vi "SIMPLE 2D Sweep -MAIN.vi"() -> ()   [LabVIEW 2025]
doc: "This is a program providing a single inclusive measurement platform in LabVIEW for every 2D sweep created by Pratap Chandra Adak."
uses:
  TYPE DEFS/S2DS_Instrument Info.ctl
  TYPE DEFS/S2DS_Instrument parameters.ctl
  TYPE DEFS/S2DS_All Channel Parameters.ctl
  TYPE DEFS/S2DS_WC info.ctl
  TYPE DEFS/S2DS_Single WC info.ctl
  TYPE DEFS/S2DS_RC info.ctl
  TYPE DEFS/S2DS_Single RC info.ctl
  TYPE DEFS/S2DS_DAC info new.ctl
  TYPE DEFS/S2DS_Single DC info.ctl
  TYPE DEFS/S2DS_Array Inst Info.ctl
  TYPE DEFS/S2DS_Sweep Info.ctl
  TYPE DEFS/S2DS_Display info.ctl
  TYPE DEFS/S2DS_Data saving info.ctl
  TYPE DEFS/S2DS_Port lists.ctl
  TYPE DEFS/S2DS_Timer.ctl
  TYPE DEFS/S2DS_WCFromFileInfo.ctl
  TYPE DEFS/S2DS_PlotInfo.ctl
  TYPE DEFS/S2DS_PlotCluster.ctl
  <vilib>/Utility/error.llb/Three Button Dialog.vi
panel:
  in  "Pause":bool
  in  "Edit Instrument?":bool
  in  "Quit sweep":bool
  out "?":string=" ( : )"
  in  "Set initial settings":bool
  out "Save location:":path
  out "Prameter error":string
  in  "Tab Control Y":enum32{"Parameters", "Additional"}(tab) caption="B(kUnit)"
  in  "Y Min":dbl caption="Min end"
  in  "Y Max":dbl=1.0 caption="Max end"
  in  "Y Bin size":dbl=0.001 caption="Data bin  size"
  in  "Y Step":dbl=0.001 caption="Ramp step size"
  in  "Y Rate up":dbl=0.1 caption="Rate up/min"
  in  "Y Rate down":dbl=0.1 caption="Rate down/min"
  in  "Y Stop at":u16(ring)=1 items=["Continue", "Stop at end", "Stop at stoppage"]
  in  "Y Skipping":u64 caption="skipping"
  in  "Y Stoppage":dbl caption="Stoppage"
  in  "Ramp Y":bool
  in  "Take data 2":u16(ring) caption="Take data" items=["in both direction", "in up direction only", "in down direction only"]
  in  "Reset skipped Y":bool
  out "Y reached":i32 caption="Reached"
  in  "Tab Control X":enum32{"Parameters", "Additional"}(tab) caption="A(TUnit)"
  in  "X Step":dbl=0.001 caption="Ramp step size"
  in  "X Rate up":dbl=0.1 caption="Rate up/min"
  in  "X Rate down":dbl=0.1 caption="Rate down/min"
  in  "X Bin size":dbl=0.001 caption="Data bin  size"
  in  "X Max":dbl=1.0 caption="Max end"
  in  "X Min":dbl caption="Min end"
  in  "Reset skipped X":bool
  in  "X Stop at":u64(ring) items=["Continue", "Stop at end", "Stop at stoppage"]
  in  "X Skipping":u64 caption="skipping"
  in  "X Stoppage":dbl caption="Stoppage"
  in  "Ramp X":bool
  in  "Take data":u16(ring) items=["in both direction", "in up direction only", "in down direction only"]
  out "X reached":i32 caption="Reached"
  in  "Hide control panel":bool
  in  "Read array instruments":bool
  in  "WC calculation":bool
  in  "Time save?":bool
  in  "Script On?":bool
  in  "Sweep":bool
  in  "Ramping":bool
  in  "Y sweep direction":bool=TRUE caption="B"
  in  "X sweep direction":bool=TRUE caption="A"
  in  "Scan type":u16(ring) items=["WC values from file", "1D Sweep in A(TUnit)", "1D Sweep in B(kUnit)", "2D Sweep in A(TUnit) within B(kUnit)", "2D Sweep in B(kUnit) within A(TUnit)"]
  out "R12":dbl caption="R9( Unit)"
  out "R13":dbl caption="R10( Unit)"
  out "X :":dbl caption="Index"
  out "Y :":dbl caption="A(TUnit)"
  out "R0":dbl caption="B(kUnit)"
  out "R1":dbl caption="R(Unit)"
  out "R2":dbl caption="Freq(Hz)"
  out "R3":dbl caption="V(V)"
  out "R4":dbl caption="R1(ohmm)"
  out "R5":dbl caption="A( Unit)"
  out "R6":dbl caption="A( Unit)"
  out "R7":dbl caption="A( Unit)"
  out "R8":dbl caption="R7( Unit)"
  out "R9":dbl caption="R8( Unit)"
  out "R10":dbl caption="R9( Unit)"
  out "R11":dbl caption="R10( Unit)"
  in  "Refresh inst info":bool
  out "Buffer length:":i32
  in  "Save now to file?":bool
  in  "Clear Buffer?":bool
  in  "Auto color":bool=TRUE
  in  "Change color?":bool
  in  "Clear plot?":bool
  in  "View Plot?":bool=TRUE
  in  "Update plot":bool=TRUE
  in  "Send email":bool
  in  "Timeout":u16=60 min=1 step=1
  in  "Export Data":bool
  in  "External control":bool
  in  "Y axis":u16(ring) items=["Index", "A(TUnit)", "B(kUnit)", "R(Unit)"]
  in  "X axis":u16(ring) items=["Index", "A(TUnit)", "B(kUnit)", "R(Unit)"]
  out "XY Graph":T1(graph) caption="Pratap"
  in  "Timer reset?":bool
  in  "Clear error?":bool
  out "Progress":i32(slide) scale=0.0..100.0
  out "Remaining time: :":string
  out "Elapsed time:":string
  out "Status":string="Back panel not set"
  # "SIMPLE 2D SWEEP (v10.3.10) ..."
  # "S"
  # "VS"
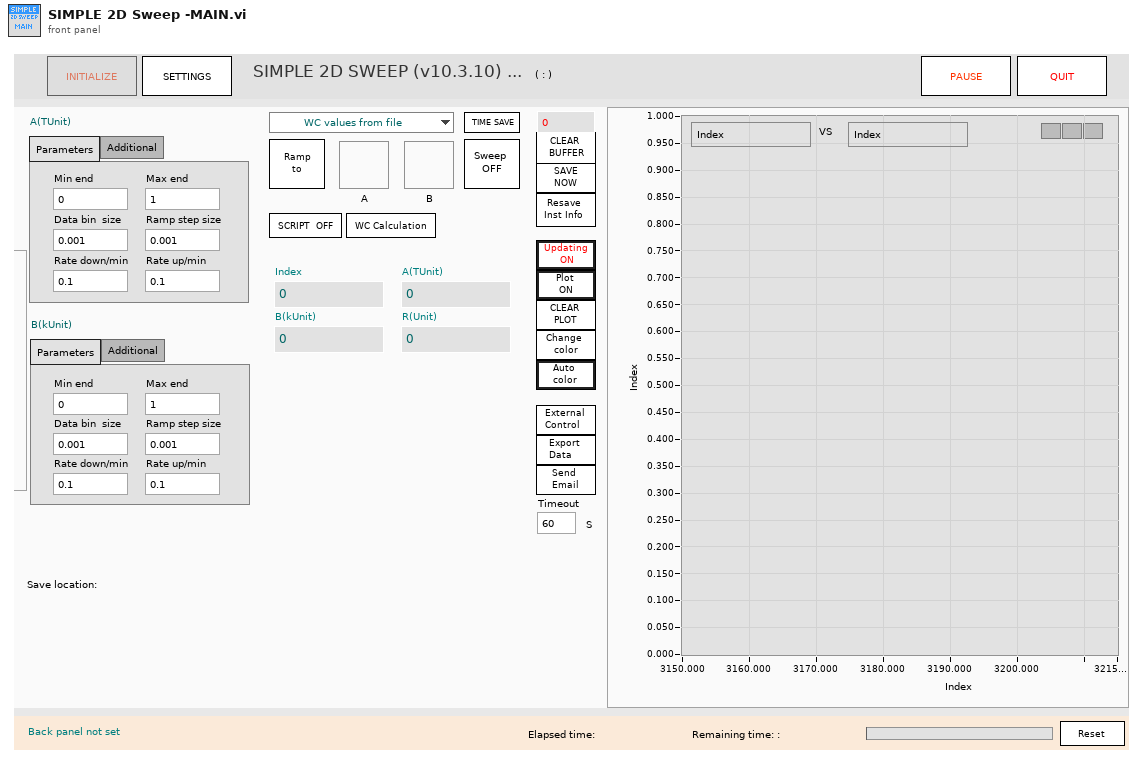
[diagram p1: front panel]
types:
  T1 = cluster{"Plot X array":dbl[], "Plot Z array":dbl[]}[]
  T2 = enum8{"Enabled", "Disabled", "Disabled and Grayed Out"}
  T3 = typedef "S2DS_Data saving info.ctl" = cluster{"File path":path, "Header":string, "File name":string, "False channel":string[][], "Channel names":string[], "Buffer size":i32, "Format":string}
  T4 = typedef "S2DS_Display info.ctl" = cluster{"WCl names with units":string[], "RC  names with units":string[], "DC  names with units":string[], "AC names with units":string[], "Indicator captions":string[], "Graph channels":string[], "Channel numbers":i32[], "User info":string}
  T5 = typedef "S2DS_All Channel Parameters.ctl" = cluster{"WC info list":T6, "RC info list":T8, "DC Info list":T10, "Array instrument info":T12, "Scan parameters":T13, "Parsed Formula Node":cluster{"Y Values":dbl[][], "Tables":i32[][][], "Variables input decode":i32[], "Variables output decode":i32[]}, "formula (in)":string}
  T6 = typedef "S2DS_WC info.ctl" = T7[]
  T7 = typedef "S2DS_Single WC info.ctl" = cluster{"Instrument identifier":string, "Write channel parameters":dbl[], "Name":string, "Unit":string}
  T8 = typedef "S2DS_RC info.ctl" = T9[]
  T9 = typedef "S2DS_Single RC info.ctl" = cluster{"Instrument identifier":string, "Factor":dbl, "Averaging":i32, "Wait (ms)":i32, "Unit":string, "Name":string}
  T10 = typedef "S2DS_DAC info new.ctl" = T11[]
  T11 = typedef "S2DS_Single DC info.ctl" = cluster{"Operation identifier":string, "DC parameters":dbl[], "U":i32, "V":i32, "Name":string, "Unit":string}
  T12 = typedef "S2DS_Array Inst Info.ctl" = cluster{"Instrument identifier":string, "Ports and units":string[][], "Factors":dbl[]}
  T13 = typedef "S2DS_Sweep Info.ctl" = cluster{"X min":ext, "X max":dbl, "Y min":dbl, "Y max":dbl, "X bin size":dbl, "Y bin size":dbl, "X stop at":dbl, "Y stop at":dbl, "X skip":u64, "Y skip":u64, "Current X":dbl, "Current Y":dbl, "X reached":i32, "Y reached":i32, "X target":dbl, "Y target":dbl, "Sweep ON?":bool, "X sweep direction":bool, "Y sweep direction":bool, "Determine X?":bool, "Determine Y?":bool, "X sweep over?":bool, "Y sweep over?":bool, "Scan type":i32, "X stopping":i32, "Y stopping":i32, "X Y Channel":u16[], "X data taking":u16, "Y data taking":u16}
  T14 = typedef "S2DS_Instrument Info.ctl" = cluster{"Instrument parameters":T15[], "DAQ Tasks":refnum<k21>[], "Total Instrument List":string[], "read inst \nVI Refnum":refnum<vi>, "type specifier Edit instruments VI Refnum":refnum<vi>, "type specifier write instrument VI Refnum (for type only)":refnum<vi>, "User instrument list":string[]}
  T15 = typedef "S2DS_Instrument parameters.ctl" = cluster{"VISA Address":refnum<visa-resource-name>, "GPIB/TCP Address":string, "String 1":string, "String 2":string, "Boolean 1":bool, "Boolean 2":bool, "Int 1":i32, "Int 2":i32, "Double 1":dbl, "Double 2":dbl}
  T16 = typedef "S2DS_Port lists.ctl" = cluster{"Write ports":string[], "Read ports":string[], "FC channels":string[][]}
  T17 = typedef "S2DS_PlotInfo.ctl" = cluster{"Plot data array":T18, "Number of curve":i32, "Present curve number XZ":i32}
  T18 = typedef "S2DS_PlotCluster.ctl" = cluster{"Plot i array":dbl[][]}[]
  T19 = typedef "S2DS_WCFromFileInfo.ctl" = cluster{"Next line to read":i32, "Next point in array":i32, "File path":path, "Data to write":dbl[][], "Read offset":i32, "Total line":i32}
  T20 = typedef "S2DS_Timer.ctl" = cluster{"Initial time ":i32, "Total step":i32, "Step completed":i32}
  T21 = cluster{"Y Values":dbl[][], "Tables":i32[][][], "Variables input decode":i32[], "Variables output decode":i32[]}
  T22 = cluster{"Plot X array":dbl[], "Plot Z1 array":dbl[]}[]
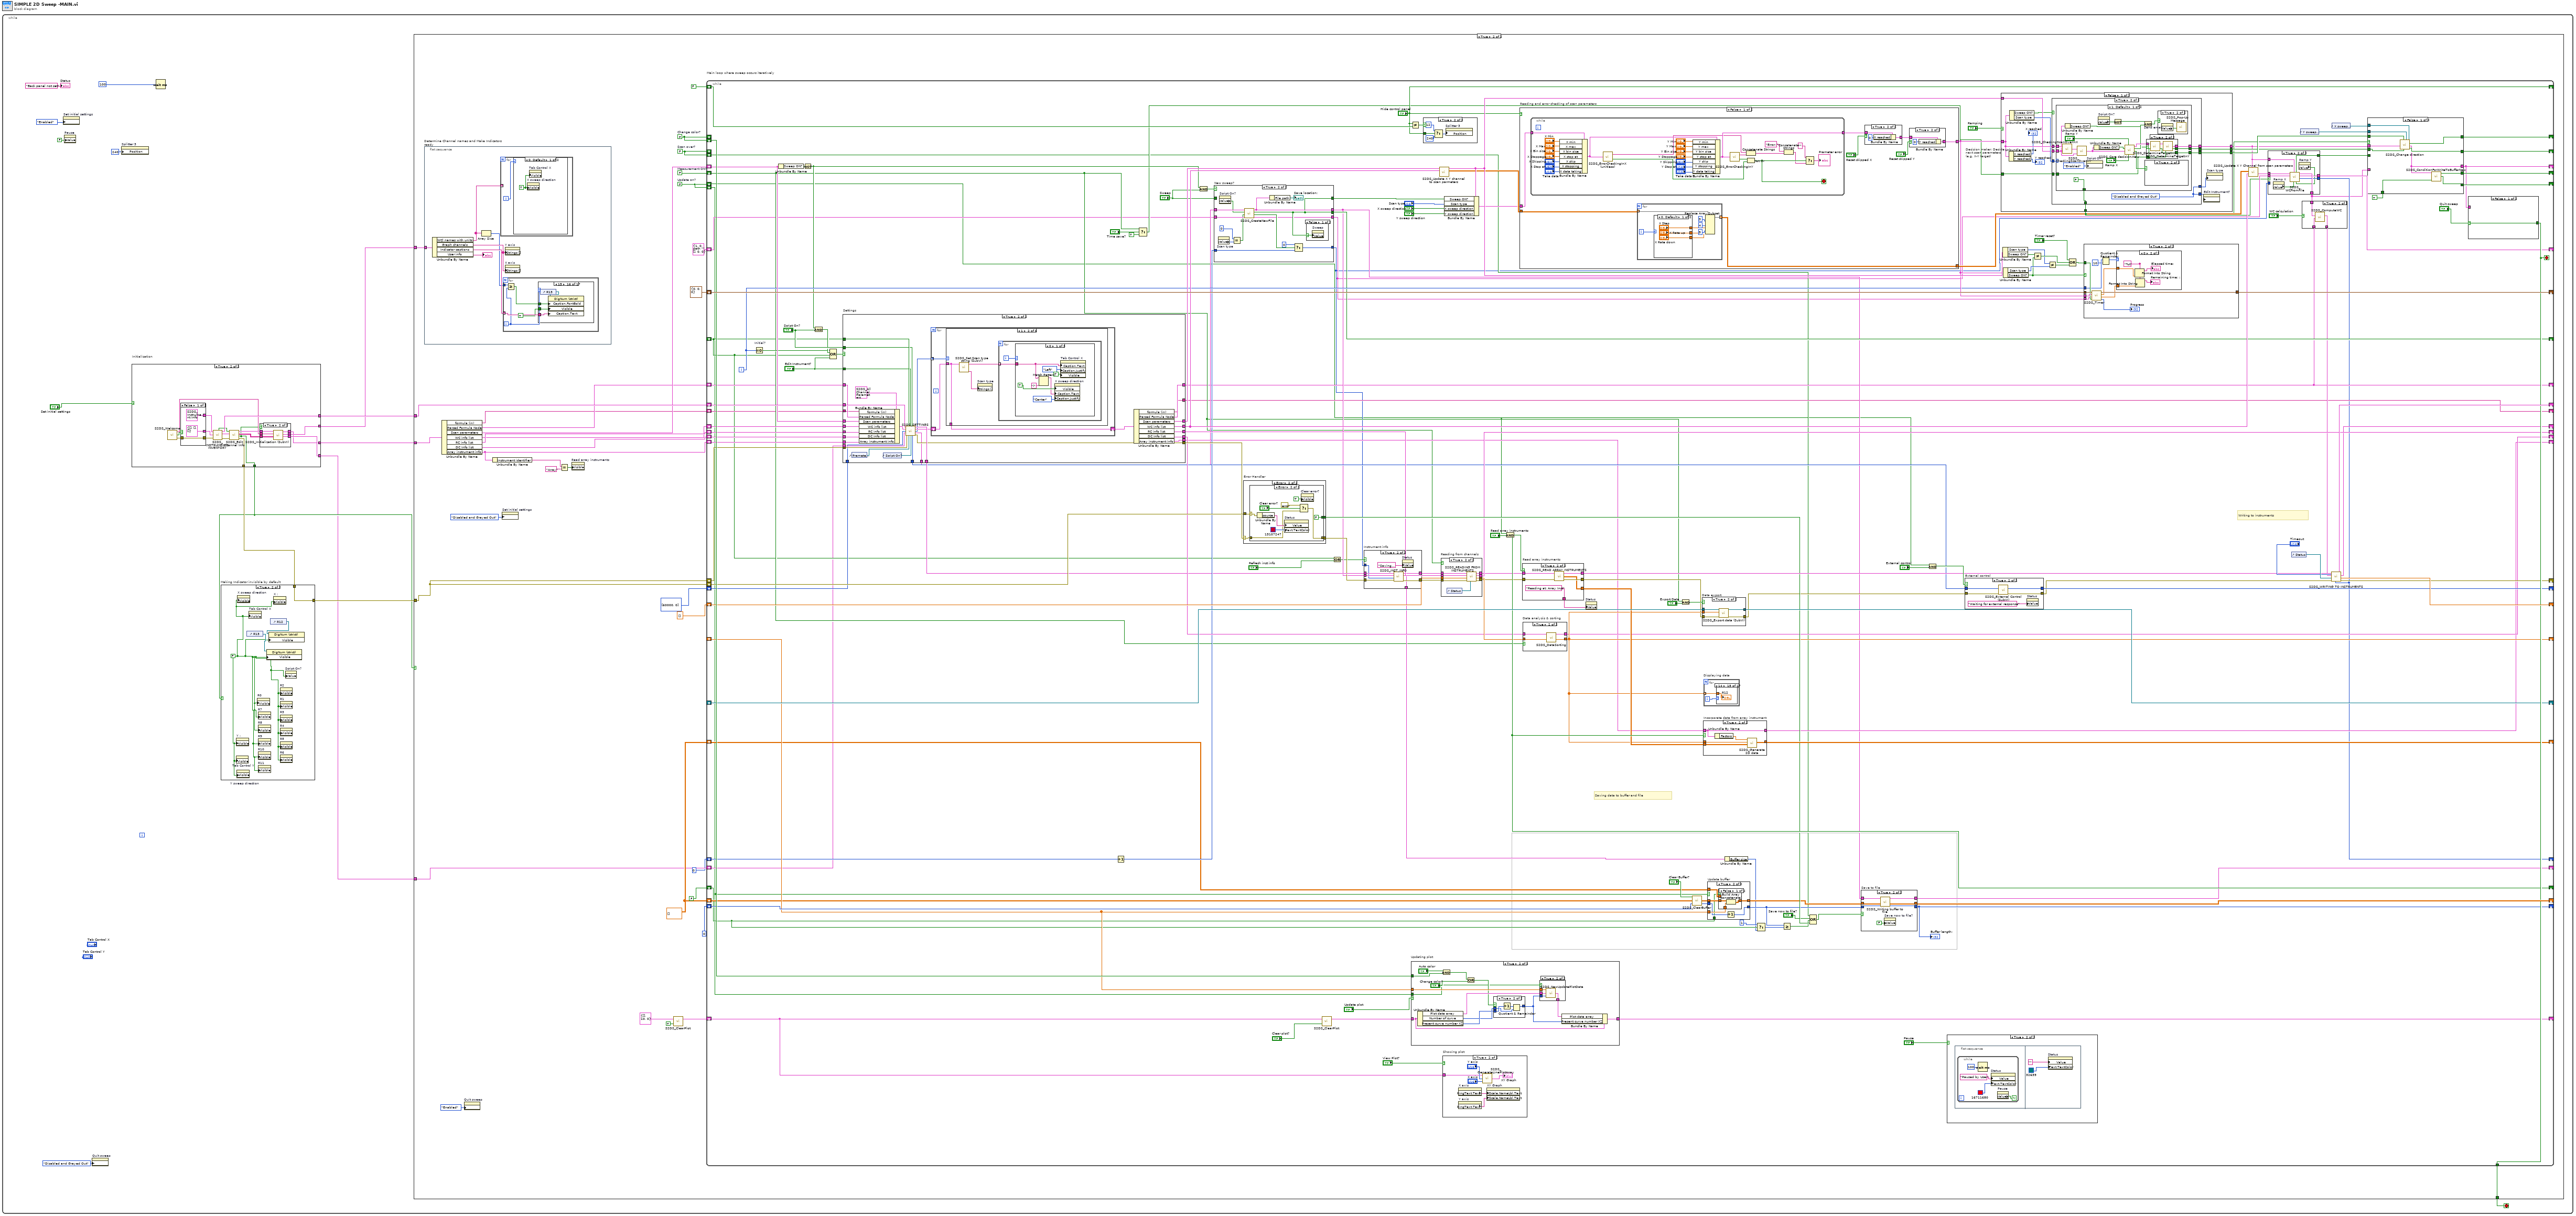
[diagram p0: block diagram]
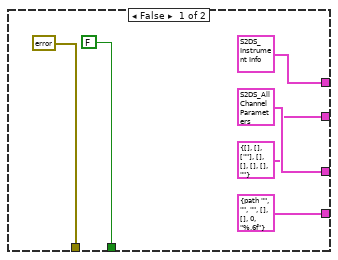
[diagram p3: hidden frame]
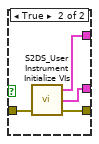
[diagram p5: hidden frame]
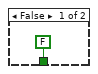
[diagram p6: hidden frame]
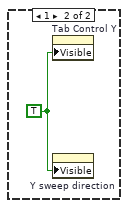
[diagram p7: hidden frame]
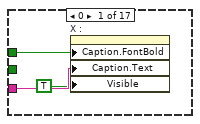
[diagram p8: hidden frame]
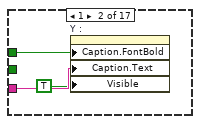
[diagram p9: hidden frame]
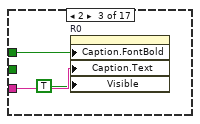
[diagram p10: hidden frame]
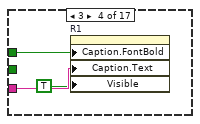
[diagram p11: hidden frame]
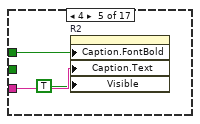
[diagram p12: hidden frame]
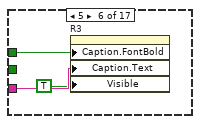
[diagram p13: hidden frame]
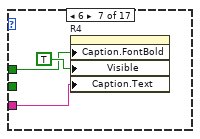
[diagram p14: hidden frame]
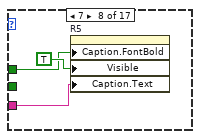
[diagram p15: hidden frame]
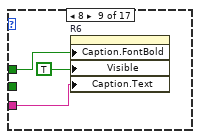
[diagram p16: hidden frame]
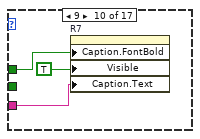
[diagram p17: hidden frame]
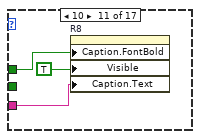
[diagram p18: hidden frame]
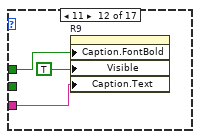
[diagram p19: hidden frame]
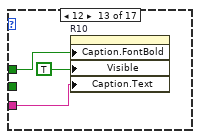
[diagram p20: hidden frame]
diagram:
  n1 = while {
    stop <- w6 stop-if-true
    n2 = property on="Set initial settings" class="Bool"("DisabledEnum"=T2."Enabled" ("Disabled")) -> ()  [unwired: 2 in, 2 out]
    n3 = property on="Pause" class="Bool (strict)"("Value"=FALSE ("Pause")) -> ()  [unwired: 2 in, 2 out]
    n4 = property on="Quit sweep" class="Bool"("DisabledEnum"=T2."Disabled and Grayed Out" ("Disabled")) -> ()  [unwired: 2 in, 2 out]
    n5 = property on="Splitter 3" class="Splitter"("Position"=240 ("Splitter Position")) -> ()  [unwired: 2 in, 2 out]
    n6 = case "Initialization" shown="True" "Set initial settings" {
      tunnel: [FALSE w29] -> w8
      tunnel: [T14 {"Instrument parameters"=[], "DAQ Tasks"=[], "Total Instrument List"=[], "read inst \nVI Refnum"=refnum, "type specifier Edit instruments VI Refnum"=refnum, "type specifier write instrument VI Refnum (for type only)"=refnum, "User instrument list"=[]} ("Instrument info (out)") w39] -> w14
      tunnel: [errorcluster {"status"=FALSE, "code"=0, "source"=""} ("error out") w43] -> w9
      tunnel: [T5 {"WC info list"=[], "RC info list"=[], "DC Info list"=[], "Array instrument info"={"Instrument identifier"="", "Ports and units"=[], "Factors"=[]}, "Scan parameters"={"X min"=0.0, "X max"=0.0, "Y min"=0.0, "Y max"=0.0, "X bin size"=0.0, "Y bin size"=0.0, "X stop at"=0.0, "Y stop at"=0.0, "X skip"=0, "Y skip"=0, "Current X"=0.0, "Current Y"=0.0, "X reached"=0, "Y reached"=0, "X target"=0.0, "Y target"=0.0, "Sweep ON?"=FALSE, "X sweep direction"=FALSE, "Y sweep direction"=FALSE, "Determine X?"=FALSE, "Determine Y?"=FALSE, "X sweep over?"=FALSE, "Y sweep over?"=FALSE, "Scan type"=0, "X stopping"=0, "Y stopping"=0, "X Y Channel"=[], "X data taking"=0, "Y data taking"=0}, "Parsed Formula Node"={"Y Values"=[], "Tables"=[], "Variables input decode"=[], "Variables output decode"=[]}, "formula (in)"=""} ("All channel parameters (out)") w30] -> w5
      tunnel: [T4 {"WCl names with units"=[], "RC  names with units"=[], "DC  names with units"=[""], "AC names with units"=[], "Indicator captions"=[], "Graph channels"=[], "Channel numbers"=[], "User info"=""} ("All channel info (Out)") w32] -> w4
      tunnel: [T3 {"File path"=path "", "Header"="", "File name"="", "False channel"=[], "Channel names"=[], "Buffer size"=0, "Format"="%.6f"} ("Data save info (out)") w31] -> w2
      frame False {
      }
      frame True {
        n7 = call "S2DS_Welcome.vi"() -> ("error out"=w36:errorcluster, "Own instrument?"=w37:bool, "User info"=w34:string[])  [unwired: 3 in]
        n8 = case shown="False" w37 {
          tunnel: [T16 {"Write ports"=[], "Read ports"=[], "FC channels"=[]} ("Port lists (out)") w57] -> w41
          tunnel: [T14 {"Instrument parameters"=[], "DAQ Tasks"=[], "Total Instrument List"=[], "read inst \nVI Refnum"=refnum, "type specifier Edit instruments VI Refnum"=refnum, "type specifier write instrument VI Refnum (for type only)"=refnum, "User instrument list"=[]} ("Instrument info (out)") w56] -> w42
          tunnel: [w53 w54] -> w40
          tunnel: w36 -> [w53 w55]
          frame False {
          }
          frame True {
            n9 = call "S2DS_User Instrument Initialize VIs.vi"("error in"=w55) -> ("error out"=w54:errorcluster, "Port lists (out)"=w57:T16, "Instrument info (out)"=w56:T14)  [unwired: 2 in]
          }
        }
        n10 = call "S2DS_INSTRUMENTS INVENTORY.vi"("Instrument Info (in)"=w42, "Port list (in)"=w41, "error in"=w40) -> ("Instrument info (out)"=w39:T14, "Port lists (out)"=w28:T16, "Error (out)"=w38:errorcluster, "Use array instrument"=w27:bool)  [unwired: 1 out]
        n11 = call "S2DS_Edit Channel Info.vi"("error in"=w38, "Port list"=w28, "Use array inst?"=w27) -> ("error out"=w43:errorcluster, "OK?"=w29:bool, "False channel (out)"=w33:string[][], "All channel parameters (out)"=w35:T5)  [unwired: 1 in]
        n12 = case shown="True" w29 {
          tunnel: [w44 w47] -> w30
          tunnel: w33 -> [_ w48]
          tunnel: [_ w50] -> w31
          tunnel: [_ w49] -> w32
          tunnel: w35 -> [w44 w45]
          tunnel: w34 -> [_ w46]
          frame False {
          }
          frame True {
            n13 = call "S2DS_Initialization (SubVI).vi"("False channel"=w48, "User info"=w46, "All channel parameters (in)"=w45) -> ("Data save info (out)"=w50:T3, "All channel info (out)"=w49:T4, "All channel parameters (out)"=w47:T5)  [unwired: 6 in]
          }
        }
      }
    }
    n14 = Wait (ms)(milliseconds to wait=u32 100) -> ()  [unwired: 1 out]
    n15 = case "Making Indicator invisible by default" shown="True" w8 {
      tunnel: [w16 w20] -> w10
      tunnel: w9 -> [w16 w20]
      frame False {
      }
      frame True {
        w17 = FALSE ("Visible")
        n16 = property on="Tab Control Y" class="TabCtl (strict)"("Visible"=w17) -> ()  [unwired: 2 in, 2 out]
        n17 = property on="Y :" class="DigNum (strict)"("Visible"=w17) -> ()  [unwired: 2 in, 2 out]
        n18 = property on="Y sweep direction" class="Bool (strict)"("Visible"=w17) -> ()  [unwired: 2 in, 2 out]
        n19 = property on="X sweep direction" class="Bool (strict)"("Visible"=w17) -> ()  [unwired: 2 in, 2 out]
        n20 = control-ref of="R13"() -> (w18:refnum<vi>)
        n21 = property on="Tab Control X" class="TabCtl (strict)"("Visible"=w17) -> ()  [unwired: 2 in, 2 out]
        n22 = property on="R0" class="DigNum (strict)"("Visible"=w17) -> ()  [unwired: 2 in, 2 out]
        n23 = property on="R7" class="DigNum (strict)"("Visible"=w17) -> ()  [unwired: 2 in, 2 out]
        n24 = property on="R8" class="DigNum (strict)"("Visible"=w17) -> ()  [unwired: 2 in, 2 out]
        n25 = property on="R9" class="DigNum (strict)"("Visible"=w17) -> ()  [unwired: 2 in, 2 out]
        n26 = property on="R10" class="DigNum (strict)"("Visible"=w17) -> ()  [unwired: 2 in, 2 out]
        n27 = property on="R11" class="DigNum (strict)"("Visible"=w17) -> ()  [unwired: 2 in, 2 out]
        n28 = property on="Property Node" class="DigNum (strict)"(reference=w18, "Visible"=w17) -> ()  [unwired: 1 in, 2 out]
        n29 = control-ref of="R12"() -> (w19:refnum<vi>)
        n30 = property on="Property Node" class="DigNum (strict)"(reference=w19, "Visible"=w17) -> ()  [unwired: 1 in, 2 out]
        n31 = property on="X :" class="DigNum (strict)"("Visible"=w17) -> ()  [unwired: 2 in, 2 out]
        n32 = property on="R2" class="DigNum (strict)"("Visible"=w17) -> ()  [unwired: 2 in, 2 out]
        n33 = property on="R1" class="DigNum (strict)"("Visible"=w17) -> ()  [unwired: 2 in, 2 out]
        n34 = property on="R3" class="DigNum (strict)"("Visible"=w17) -> ()  [unwired: 2 in, 2 out]
        n35 = property on="R4" class="DigNum (strict)"("Visible"=w17) -> ()  [unwired: 2 in, 2 out]
        n36 = property on="R5" class="DigNum (strict)"("Visible"=w17) -> ()  [unwired: 2 in, 2 out]
        n37 = property on="R6" class="DigNum (strict)"("Visible"=w17) -> ()  [unwired: 2 in, 2 out]
        n38 = property on="Script On?" class="Bool (strict)"("Value"=w17) -> ()  [unwired: 2 in, 2 out]
      }
    }
    n39 = case shown="True" w8 {
      tunnel: w14 -> [_ w92]
      tunnel: w10 -> [_ w76]
      tunnel: [FALSE ("Yes, exit.") w88] -> w6
      tunnel: w5 -> [_ w80]
      tunnel: w4 -> [_ w79]
      tunnel: w2 -> [_ w71]
      frame False {
      }
      frame True {
        w74 = FALSE  # Change color?
        w86 = FALSE  # Scan over?
        w77 = FALSE  # Update on?
        w89 = FALSE  # Measurement ON?
        w78 = dbl[][] [] ("Data array out")
        n40 = flat-sequence "Determine Channel names and Make Indicators ready" {
          tunnel: w79 -> [w98]
          frame #0 {
            n41 = Unbundle By Name(w98) -> ("WCl names with units"=w94:string[], "Graph channels"=w97:string[], "Indicator captions"=w96:string[], "User info"=→"?":string)
            n42 = Array Size(array=w94) -> (size(s)=w93:i32)
            n43 = for {
              tunnel: w94 -> [_] mode=indexing
              i -> [w99]
              n44 = case shown="0, Default" w99 {
                frame 0, Default {
                  w100 = TRUE ("Visible")
                  n45 = property on="X sweep direction" class="Bool (strict)"("Visible"=w100) -> ()  [unwired: 2 in, 2 out]
                  n46 = property on="Tab Control X" class="TabCtl (strict)"("Visible"=w100) -> ()  [unwired: 2 in, 2 out]
                }
                frame 1 {
                  w101 = TRUE ("Visible")
                  n47 = property on="Tab Control Y" class="TabCtl (strict)"("Visible"=w101) -> ()  [unwired: 2 in, 2 out]
                  n48 = property on="Y sweep direction" class="Bool (strict)"("Visible"=w101) -> ()  [unwired: 2 in, 2 out]
                }
              }
            }
            n49 = for {
              tunnel: w96 -> [w106] mode=indexing
              tunnel: w93 -> [w105]
              i -> [w104]
              n50 = Greater Or Equal?(x=w105, y=w104) -> (x >= y?=w103:bool)
              n51 = case shown="15" w104 {
                tunnel: w106 -> [w109 w112 w115 w118 w121 w124 w127 w129 w132 w135 w139 w142 w145 w148 w151 w155 _]
                tunnel: w103 -> [w107 w110 w113 w116 w119 w122 w125 w128 w131 w134 w137 w140 w143 w146 w152 w156 _]
                tunnel: TRUE ("Visible") -> [_ _ _ _ _ _ _ _ _ _ _ _ _ _ w150 w154 _]
                frame 0 {
                  n52 = property on="X :" class="DigNum (strict)"("Caption.FontBold"=w107, "Caption.Text"=w109, "Visible"=TRUE) -> ()  [unwired: 2 in, 2 out]
                }
                frame 1 {
                  n53 = property on="Y :" class="DigNum (strict)"("Caption.FontBold"=w110, "Caption.Text"=w112, "Visible"=TRUE) -> ()  [unwired: 2 in, 2 out]
                }
                frame 2 {
                  n54 = property on="R0" class="DigNum (strict)"("Caption.FontBold"=w113, "Caption.Text"=w115, "Visible"=TRUE) -> ()  [unwired: 2 in, 2 out]
                }
                frame 3 {
                  n55 = property on="R1" class="DigNum (strict)"("Caption.FontBold"=w116, "Caption.Text"=w118, "Visible"=TRUE) -> ()  [unwired: 2 in, 2 out]
                }
                frame 4 {
                  n56 = property on="R2" class="DigNum (strict)"("Caption.FontBold"=w119, "Caption.Text"=w121, "Visible"=TRUE) -> ()  [unwired: 2 in, 2 out]
                }
                frame 5 {
                  n57 = property on="R3" class="DigNum (strict)"("Caption.FontBold"=w122, "Caption.Text"=w124, "Visible"=TRUE) -> ()  [unwired: 2 in, 2 out]
                }
                frame 6 {
                  n58 = property on="R4" class="DigNum (strict)"("Caption.FontBold"=w125, "Visible"=TRUE, "Caption.Text"=w127) -> ()  [unwired: 2 in, 2 out]
                }
                frame 7 {
                  n59 = property on="R5" class="DigNum (strict)"("Caption.FontBold"=w128, "Visible"=TRUE, "Caption.Text"=w129) -> ()  [unwired: 2 in, 2 out]
                }
                frame 8 {
                  n60 = property on="R6" class="DigNum (strict)"("Caption.FontBold"=w131, "Visible"=TRUE, "Caption.Text"=w132) -> ()  [unwired: 2 in, 2 out]
                }
                frame 9 {
                  n61 = property on="R7" class="DigNum (strict)"("Caption.FontBold"=w134, "Visible"=TRUE, "Caption.Text"=w135) -> ()  [unwired: 2 in, 2 out]
                }
                frame 10 {
                  n62 = property on="R8" class="DigNum (strict)"("Caption.FontBold"=w137, "Visible"=TRUE, "Caption.Text"=w139) -> ()  [unwired: 2 in, 2 out]
                }
                frame 11 {
                  n63 = property on="R9" class="DigNum (strict)"("Caption.FontBold"=w140, "Visible"=TRUE, "Caption.Text"=w142) -> ()  [unwired: 2 in, 2 out]
                }
                frame 12 {
                  n64 = property on="R10" class="DigNum (strict)"("Caption.FontBold"=w143, "Visible"=TRUE, "Caption.Text"=w145) -> ()  [unwired: 2 in, 2 out]
                }
                frame 13 {
                  n65 = property on="R11" class="DigNum (strict)"("Caption.FontBold"=w146, "Visible"=TRUE, "Caption.Text"=w148) -> ()  [unwired: 2 in, 2 out]
                }
                frame 14 {
                  n66 = control-ref of="R12"() -> (w149:refnum<vi>)
                  n67 = property on="Property Node" class="DigNum (strict)"(reference=w149, "Caption.FontBold"=w152, "Visible"=w150, "Caption.Text"=w151) -> ()  [unwired: 1 in, 2 out]
                }
                frame 15 {
                  n68 = control-ref of="R13"() -> (w153:refnum<vi>)
                  n69 = property on="Property Node" class="DigNum (strict)"(reference=w153, "Caption.FontBold"=w156, "Visible"=w154, "Caption.Text"=w155) -> ()  [unwired: 1 in, 2 out]
                }
                frame 16, Default {
                }
              }
            }
            n70 = property on="Y axis" class="Ring (strict)"("Strings []"=w97) -> ()  [unwired: 2 in, 2 out]
            n71 = property on="X axis" class="Ring (strict)"("Strings []"=w97) -> ()  [unwired: 2 in, 2 out]
          }
        }
        n72 = Unbundle By Name(w80) -> ("formula (in)"=w64:string, "Parsed Formula Node"=w65:T21, "Scan parameters"=w70:T13, "WC info list"=w81:T6, "RC info list"=w82:T8, "DC Info list"=w83:T10, "Array instrument info"=w66:T12)
        n73 = property on="Quit sweep" class="Bool"("DisabledEnum"=T2."Enabled" ("Disabled")) -> ()  [unwired: 2 in, 2 out]
        n74 = Unbundle By Name(w66) -> ("Instrument identifier"=w67:string)
        n75 = property on="Set initial settings" class="Bool"("DisabledEnum"=T2."Disabled and Grayed Out" ("Disabled")) -> ()  [unwired: 2 in, 2 out]
        n76 = Equal?(x=w67, y="Array") -> (x = y?=w59:bool)
        n77 = property on="Read array instruments" class="Bool (strict)"("Visible"=w59) -> ()  [unwired: 2 in, 2 out]
        n78 = call "S2DS_ClearPlot.vi"("Clear plot?"=TRUE, "Cluster in"=T17 {"Plot data array"=[], "Number of curve"=10, "Present curve number XZ"=0}) -> ("Cluster out"=w61:T17)  [unwired: 1 in]
        n79 = while "Main loop where sweep occurs iteratively" {
          shift-right: [w242] -> _
          shift-left: w71 -> [w160]
          shift-right: [w166] -> _
          shift-left: w61 -> [w309]
          shift-right: [w312] -> _
          shift-left: T20 {"Initial time "=0, "Total step"=0, "Step completed"=0} ("Timer Cluster in") -> [w310]
          shift-right: [w193] -> _
          shift-left: w70 -> [w232]
          shift-right: [w204] -> _
          shift-left: w81 -> [w300]
          shift-right: [w311] -> _
          shift-left: w92 -> [w239]
          shift-right: [w292] -> _
          shift-left: w76 -> [w237]
          shift-right: [w308] -> _
          shift-left: dbl[] [] ("Data out") -> [w246]
          shift-right: [w243] -> _
          shift-left: w82 -> [w241]
          shift-right: [w307] -> _
          shift-left: w78 -> [w215]
          shift-right: [w299] -> _
          shift-left: 0 -> [w298]
          shift-right: [w306] -> _
          shift-left: w74 -> [_]
          shift-right: [w245] -> _
          shift-left: _ -> [w244]
          shift-right: [w304] -> _
          shift-left: w89 -> [w191]
          shift-right: [w303] -> _
          shift-left: w77 -> [w158]
          shift-left: w77 -> [w157]
          shift-left: w74 -> [w305]
          shift-right: [w302] -> _
          shift-left: w86 -> [_]
          shift-left: w86 -> [w169]
          tunnel: [w301] -> w88
          shift-right: [w297] -> _
          shift-left: i32[] [60000, 0] -> [w212]
          shift-right: [w296] -> _
          shift-left: _ -> [w295]
          shift-right: [w294] -> _
          shift-left: FALSE ("Change color") -> [w213]
          shift-right: [w293] -> _
          shift-left: w78 -> [w214]
          shift-left: w76 -> [w291]
          shift-right: ["Hide control panel"] -> _
          shift-left: FALSE ("Hide control panel") -> [w251]
          shift-right: [w234] -> _
          shift-left: w83 -> [w236]
          shift-right: [w201] -> _
          shift-left: _ -> [w165]
          shift-right: [w177] -> _
          shift-left: 0 -> [w225]
          shift-right: [w205] -> _
          shift-left: w66 -> [w207]
          shift-right: [w181] -> _
          shift-left: w65 -> [w182]
          shift-right: [w179] -> _
          shift-left: w64 -> [w180]
          shift-right: [w176] -> _
          shift-left: T19 {"Next line to read"=1, "Next point in array"=0, "File path"=path "", "Data to write"=[], "Read offset"=0, "Total line"=0} ("WC read from file info (out)") -> [w175]
          i -> [w226]
          stop <- w301 stop-if-true
          # "Saving data to buffer and file"
          # "Writing to instruments"
          n80 = Equal To 0? "Initial?"(x=w226) -> (x = 0?=w195:bool)
          n81 = Unbundle By Name(w232) -> ("Sweep ON?"=w231:bool)
          n82 = Not(x=w231) -> (.not. x?=w200:bool)
          n83 = And(x=w200, y="Script On?") -> (x .and. y?=w228:bool)
          n84 = Compound Arithmetic op=OR(w195, w228, w165, "Edit Instrument?") -> (w227:bool)
          n85 = case "Settings" shown="True" w227 {
            tunnel: [w430 w449] -> w230
            tunnel: w300 -> [w430 w445]
            tunnel: w241 -> [w429 w444]
            tunnel: [w429 w448] -> w240
            tunnel: w239 -> [w428 w462]
            tunnel: [w428 w461] -> w219
            tunnel: [w427 w459] -> w238
            tunnel: w237 -> [w427 w460]
            tunnel: w236 -> [w426 w443]
            tunnel: [w426 w447] -> w235
            tunnel: w232 -> [w425 w446]
            tunnel: [w425 w450] -> w233
            tunnel: [w424 w457] -> w198
            tunnel: w160 -> [w424 w458]
            tunnel: "Edit Instrument?" -> [_ w440]
            tunnel: "Script On?" -> [_ w439]
            tunnel: w165 -> [_ w441]
            tunnel: w212 -> [w423 w438]
            tunnel: [w423 w437] -> w211
            tunnel: w207 -> [w422 w436]
            tunnel: [w422 w435] -> w206
            tunnel: [w421 w433] -> w181
            tunnel: w182 -> [w421 w434]
            tunnel: w180 -> [w420 w432]
            tunnel: [w420 w431] -> w179
            frame False {
            }
            frame True {
              n86 = control-ref of="Prameter error"() -> (w454:refnum<vi>)
              n87 = Bundle By Name(cluster=T5 {"WC info list"=[], "RC info list"=[], "DC Info list"=[], "Array instrument info"={"Instrument identifier"="", "Ports and units"=[], "Factors"=[]}, "Scan parameters"={"X min"=0.0, "X max"=0.0, "Y min"=0.0, "Y max"=0.0, "X bin size"=0.0, "Y bin size"=0.0, "X stop at"=0.0, "Y stop at"=0.0, "X skip"=0, "Y skip"=0, "Current X"=0.0, "Current Y"=0.0, "X reached"=0, "Y reached"=0, "X target"=0.0, "Y target"=0.0, "Sweep ON?"=FALSE, "X sweep direction"=FALSE, "Y sweep direction"=FALSE, "Determine X?"=FALSE, "Determine Y?"=FALSE, "X sweep over?"=FALSE, "Y sweep over?"=FALSE, "Scan type"=0, "X stopping"=0, "Y stopping"=0, "X Y Channel"=[], "X data taking"=0, "Y data taking"=0}, "Parsed Formula Node"={"Y Values"=[], "Tables"=[], "Variables input decode"=[], "Variables output decode"=[]}, "formula (in)"=""} ("All channel parameters"), "formula (in)"=w432, "Parsed Formula Node"=w434, "Scan parameters"=w446, "WC info list"=w445, "RC info list"=w444, "DC Info list"=w443, "Array instrument info"=w436) -> (w455:T5)
              n88 = control-ref of="Script On?"() -> (w453:refnum<vi>)
              n89 = call "S2DS_SETTINGS.vi"("Instrument Info (out) in"=w462, "New sweep?"=w441, "Manual instruction?"=w440, "Script on?"=w439, "All channel parameters"=w455, "External control settings"=w438, "Data save info (in)"=w458, "error in (no error)"=w460, "Prameter error"=w454, "Script On?"=w453) -> ("Instrument Info (out) out"=w461:T14, "All channel parameters (out)"=w452:T5, "Update instruction"=w442:i32[], "Data save info (out)"=w457:T3, "External control settings out"=w437:i32[], "error out"=w459:errorcluster)
              n90 = for {
                shift-right: [w464] -> w451
                shift-left: w452 -> [w465]
                tunnel: w442 -> [w463] mode=indexing
                n91 = case shown="1" w463 {
                  tunnel: w465 -> [w466 w467 w485 w490 w497 w507]
                  tunnel: [w466 w467 w485 w490 w497 w507] -> w464
                  frame 0, Default {
                  }
                  frame 1 {
                    n92 = call "S2DS_Set Scan type string (SubVI).vi"("All channel parameters (in)"=w467) -> ("Scan type string"=w468:string[], "X Y Channel names (out)"=w469:string[])  [unwired: 9 in]
                    n93 = property on="Scan type" class="Ring (strict)"("Strings []"=w468) -> ()  [unwired: 2 in, 2 out]
                    n94 = for {
                      tunnel: w469 -> [w470] mode=indexing
                      i -> [w471]
                      n95 = case shown="0" w471 {
                        tunnel: w470 -> [w473 w480 _]
                        frame 0 {
                          n96 = Match Pattern(string=w473, regular expression="(") -> (before substring=w472:string)  [unwired: 1 in, 3 out]
                          n97 = property on="X sweep direction" class="Bool (strict)"("Visible"=TRUE, "Caption.Text"=w472, "Caption.Justify"=enum16{"Left", "Center", "Right"}."Center" ("Caption.Justification")) -> ()  [unwired: 2 in, 2 out]
                          n98 = property on="Tab Control X" class="TabCtl (strict)"("Caption.Text"=w473, "Caption.Justify"=enum16{"Left", "Center", "Right"}."Left" ("Caption.Justification"), "Visible"=TRUE) -> ()  [unwired: 2 in, 2 out]
                        }
                        frame 1 {
                          w483 = TRUE ("Visible")
                          n99 = Match Pattern(string=w480, regular expression="(") -> (before substring=w479:string)  [unwired: 1 in, 3 out]
                          n100 = property on="Y sweep direction" class="Bool (strict)"("Visible"=w483, "Caption.Text"=w479, "Caption.Justify"=enum16{"Left", "Center", "Right"}."Center" ("Caption.Justification")) -> ()  [unwired: 2 in, 2 out]
                          n101 = property on="Tab Control Y" class="TabCtl (strict)"("Caption.Text"=w480, "Caption.Justify"=enum16{"Left", "Center", "Right"}."Left" ("Caption.Justification"), "Visible"=w483) -> ()  [unwired: 2 in, 2 out]
                        }
                        frame 2, Default {
                        }
                      }
                    }
                  }
                  frame 2 {
                    n102 = Unbundle By Name(w485) -> ("Scan parameters.Sweep ON?"=w486:bool, "Scan parameters.X sweep direction"=w487:bool, "Scan parameters.Y sweep direction"=w488:bool, "Scan parameters.Scan type"=w489:i32)
                    n103 = property on="Sweep" class="Bool (strict)"("Value"=w486) -> ()  [unwired: 2 in, 2 out]
                    n104 = property on="X sweep direction" class="Bool (strict)"("Value"=w487) -> ()  [unwired: 2 in, 2 out]
                    n105 = property on="Y sweep direction" class="Bool (strict)"("Value"=w488) -> ()  [unwired: 2 in, 2 out]
                    n106 = property on="Scan type" class="Ring (strict)"("Value"=w489) -> ()  [unwired: 2 in, 2 out]
                  }
                  frame 3 {
                    n107 = Unbundle By Name(w490) -> ("Scan parameters.X min"=w491:ext, "Scan parameters.X max"=w492:dbl, "Scan parameters.X bin size"=w493:dbl, "Scan parameters.X stop at"=w494:dbl, "Scan parameters.X stopping"=w496:i32, "Scan parameters.X skip"=w495:u64)
                    n108 = property on="X Min" class="DigNum (strict)"("Value"=w491) -> ()  [unwired: 2 in, 2 out]
                    n109 = property on="X Max" class="DigNum (strict)"("Value"=w492) -> ()  [unwired: 2 in, 2 out]
                    n110 = property on="X Bin size" class="DigNum (strict)"("Value"=w493) -> ()  [unwired: 2 in, 2 out]
                    n111 = property on="X Stoppage" class="DigNum (strict)"("Value"=w494) -> ()  [unwired: 2 in, 2 out]
                    n112 = property on="X Stop at" class="Ring (strict)"("Value"=w496) -> ()  [unwired: 2 in, 2 out]
                    n113 = property on="X Skipping" class="DigNum (strict)"("Value"=w495) -> ()  [unwired: 2 in, 2 out]
                  }
                  frame 4 {
                    n114 = Unbundle By Name(w497) -> ("Scan parameters.Y min"=w498:dbl, "Scan parameters.Y max"=w499:dbl, "Scan parameters.Y bin size"=w500:dbl, "Scan parameters.Y stop at"=w501:dbl, "Scan parameters.Y stopping"=w503:i32, "Scan parameters.Y skip"=w502:u64)
                    n115 = property on="Y Min" class="DigNum (strict)"("Value"=w498) -> ()  [unwired: 2 in, 2 out]
                    n116 = property on="Y Max" class="DigNum (strict)"("Value"=w499) -> ()  [unwired: 2 in, 2 out]
                    n117 = property on="Y Bin size" class="DigNum (strict)"("Value"=w500) -> ()  [unwired: 2 in, 2 out]
                    n118 = property on="Y Stoppage" class="DigNum (strict)"("Value"=w501) -> ()  [unwired: 2 in, 2 out]
                    n119 = property on="Y Stop at" class="Ring (strict)"("Value"=w503) -> ()  [unwired: 2 in, 2 out]
                    n120 = property on="Y Skipping" class="DigNum (strict)"("Value"=w502) -> ()  [unwired: 2 in, 2 out]
                  }
                  frame 5 {
                    n121 = Unbundle By Name(w507) -> ("Scan parameters"=w505:T13, "WC info list"=w506:T6)
                    n122 = call "S2DS_Update X Y channel to scan parmeters.vi"("Write channel info in"=w506, "Sweep info in"=w505) -> ("Write channel parameters (out)"=w504:dbl[][])  [unwired: 8 in, 1 out]
                    n123 = for {
                      tunnel: w504 -> [w514] mode=indexing
                      i -> [w515]
                      n124 = Index Array(array=w514, index #1=3 ("index"), index #2=4 ("index"), index #3=5 ("index")) -> (element #1=w510:dbl, element #2=w509:dbl, element #3=w508:dbl)
                      n125 = case shown="0, Default" w515 {
                        tunnel: w510 -> [w518 w521]
                        tunnel: w509 -> [w517 w520]
                        tunnel: w508 -> [w516 w519]
                        frame 0, Default {
                          n126 = property on="X Step" class="DigNum (strict)"("Value"=w518) -> ()  [unwired: 2 in, 2 out]
                          n127 = property on="X Rate up" class="DigNum (strict)"("Value"=w517) -> ()  [unwired: 2 in, 2 out]
                          n128 = property on="X Rate down" class="DigNum (strict)"("Value"=w516) -> ()  [unwired: 2 in, 2 out]
                        }
                        frame 1 {
                          n129 = property on="Y Step" class="DigNum (strict)"("Value"=w521) -> ()  [unwired: 2 in, 2 out]
                          n130 = property on="Y Rate up" class="DigNum (strict)"("Value"=w520) -> ()  [unwired: 2 in, 2 out]
                          n131 = property on="Y Rate down" class="DigNum (strict)"("Value"=w519) -> ()  [unwired: 2 in, 2 out]
                        }
                      }
                    }
                  }
                }
              }
              n132 = Unbundle By Name(w451) -> ("formula (in)"=w431:string, "Parsed Formula Node"=w433:T21, "Scan parameters"=w450:T13, "WC info list"=w449:T6, "RC info list"=w448:T8, "DC Info list"=w447:T10, "Array instrument info"=w435:T12)
            }
          }
          n133 = Increment(x=w225) -> (x+1=w224:i32)
          n134 = Select(t=w191, s="Time save?", f=TRUE) -> (s? t:f=w190:bool)
          n135 = And(x=w200, y="Sweep") -> (x .and. y?=w222:bool)
          n136 = case "New sweep?" shown="True" w222 {
            selector: w222 -> [w675 _]
            tunnel: w198 -> [w678 w692]
            tunnel: [w678 w691] -> w197
            tunnel: w224 -> [w677 w686]
            tunnel: [w677 w688] -> w161
            tunnel: [w676 w683] -> w202
            tunnel: "Sweep" -> [w676 _]
            tunnel: [w675 w683] -> w201
            tunnel: w175 -> [w674 w684]
            tunnel: [w674 w682] -> w168
            frame False {
            }
            frame True {
              n137 = property on="Scan type" class="Ring (strict)"() -> ("Value"=w681:u16)  [unwired: 2 in, 2 out]
              n138 = property on="Script On?" class="Bool (strict)"() -> ("Value"=w689:bool)  [unwired: 2 in, 2 out]
              n139 = Equal?(x=u16 0, y=w681) -> (x = y?=w679:bool)
              n140 = call "S2DS_CreateNewFile.vi"("WC read from file info (in)"=w684, "WC from file?"=w679, "Script on?"=w689, "File info"=w692) -> ("WC read from file info (out)"=w682:T19, "Overwrite or create new file?"=w685:bool, "Sweep continue?"=w683:bool, "File info (out)"=w691:T3)
              n141 = Unbundle By Name(w691) -> ("File path"=→"Save location:":path)
              n142 = Select(t=0, s=w685, f=w686) -> (s? t:f=w688:i32)
              n143 = case shown="False" w683 {
                selector: w683 -> [w693 _]
                frame False {
                  n144 = property on="Sweep" class="Bool (strict)"("Value"=w693) -> ()  [unwired: 2 in, 2 out]
                }
                frame True {
                }
              }
            }
          }
          n145 = case "Error Handler" shown="Error" w238 {
            selector: w238 -> [w736 w740]
            tunnel: [w736 w739] -> w217
            tunnel: w291 -> [_ w738]
            tunnel: [FALSE ("Save now to file?") w737] -> w281
            frame No Error {
              n146 = property on="Status" class="Str"("Text.TextColor"=u32 32639) -> ()  [unwired: 2 in, 2 out]
              n147 = property on="Clear error?" class="Bool"("Visible"=FALSE) -> ()  [unwired: 2 in, 2 out]
            }
            frame Error {
              n148 = case shown="Error" w738 {
                selector: w738 -> [_ w755]
                tunnel: w740 -> [w745 w751]
                tunnel: [w744 w750] -> w739
                tunnel: [TRUE ("Save now to file?") FALSE ("Save now to file?")] -> w737
                frame No Error {
                  n149 = call "S2DS_Error Pop-Up.vi"("error constant"=w745, "Send mail?"="Send email") -> ("error constant (out)"=w744:errorcluster, "Stop sweep?"=w743:bool)  [unwired: 8 in]
                  n150 = case shown="True" w743 {
                    frame False {
                    }
                    frame True {
                      n151 = property on="Sweep" class="Bool (strict)"("Value"=FALSE) -> ()  [unwired: 2 in, 2 out]
                    }
                  }
                }
                frame Error {
                  n152 = Unbundle By Name(w755) -> ("source"=w754:string)
                  n153 = property on="Status" class="Str"("Value"=w754, "Text.TextColor"=u32 13107247) -> ()  [unwired: 2 in, 2 out]
                  n154 = Select(t=errorcluster {"status"=FALSE, "code"=0, "source"=""}, s="Clear error?", f=w751) -> (s? t:f=w750:errorcluster)
                  n155 = property on="Clear error?" class="Bool"("Visible"=TRUE) -> ()  [unwired: 2 in, 2 out]
                }
              }
            }
          }
          n156 = call "S2DS_ClearPlot.vi"("Clear plot?"="Clear plot?", "Cluster in"=w309) -> ("Cluster out"=w185:T17)  [unwired: 1 in]
          n157 = Or(x=w165, y="Refresh inst info") -> (x .or. y?=w163:bool)
          n158 = case "Instrument info" shown="True" w163 {
            tunnel: [w385 w393] -> w218
            tunnel: w219 -> [w385 w392]
            tunnel: [w384 w391] -> w216
            tunnel: w217 -> [w384 w390]
            tunnel: [w383 w389] -> w196
            tunnel: w197 -> [w383 w388]
            tunnel: w161 -> [_ w386]
            frame False {
            }
            frame True {
              n159 = call "S2DS_INST_INFO.vi"("error in (no error)"=w390, "Index"=w386, "Data save info in"=w388, "Instrument Info in"=w392) -> ("error out"=w391:errorcluster, "Data save info out"=w389:T3, "Instrument Info out"=w393:T14)  [unwired: 5 in]
              n160 = property on="Status" class="Str"("Value"="Saving instrument information" ("Status")) -> ()  [unwired: 2 in, 2 out]
            }
          }
          n161 = Not Equal?(x="Hide control panel", y=w251) -> (x != y?=w249:bool)
          n162 = case "Updating plot" shown="True" "Update plot" {
            tunnel: w185 -> [w352 w366]
            tunnel: [w352 w364] -> w166
            tunnel: w244 -> [_ w359]
            tunnel: w305 -> [_ w357]
            tunnel: w157 -> [_ w353]
            frame False {
            }
            frame True {
              n163 = Unbundle By Name(w366) -> ("Plot data array"=w361:T18, "Number of curve"=w362:i32, "Present curve number XZ"=w363:i32)
              n164 = And(x="Auto color", y=w357) -> (x .and. y?=w356:bool)
              n165 = Or(x=w356, y="Change color?") -> (x .or. y?=w354:bool)
              n166 = case shown="True" w354 {
                tunnel: w363 -> [w372 w376]
                tunnel: [w372 w374] -> w358
                tunnel: w362 -> [_ w373]
                frame False {
                }
                frame True {
                  n167 = Increment(x=w376) -> (x+1=w375:i32)
                  n168 = Quotient & Remainder(x=w375, y=w373) -> (x-y*floor(x/y)=w374:i32)  [unwired: 1 out]
                }
              }
              n169 = case shown="True" w353 {
                tunnel: w361 -> [w367 w371]
                tunnel: [w367 w370] -> w360
                tunnel: w359 -> [_ w369]
                tunnel: w358 -> [_ w368]
                frame False {
                }
                frame True {
                  n170 = call "S2DS_NewUpdatePlotData.vi"("Present curve number XZ"=w368, "Plot data array"=w371, "Data"=w369) -> ("Plot data array out"=w370:T18)  [unwired: 2 in]
                }
              }
              n171 = Bundle By Name(cluster=w366, "Plot data array"=w360, "Present curve number XZ"=w358) -> (w364:T17)
            }
          }
          n172 = case shown="True" w249 {
            tunnel: "Hide control panel" -> [_ w419]
            frame False {
            }
            frame True {
              n173 = Select(t=12 ("Splitter Position"), s=w419, f=240) -> (s? t:f=w416:i32)
              n174 = property on="Splitter 3" class="Splitter"("Position"=w416) -> ()  [unwired: 2 in, 2 out]
            }
          }
          n175 = call "S2DS_Update X Y channel to scan parmeters.vi"("Write channel info in"=w230, "Sweep info in"=w233) -> ("Write channel parameters (out)"=w267:dbl[][], "Sweep info out"=w280:T13)  [unwired: 8 in]
          n176 = case "Reading from channels" shown="True" w191 {
            tunnel: [w776 w782] -> w289
            tunnel: w216 -> [w778 w786]
            tunnel: [w778 w785] -> w220
            tunnel: w218 -> [w777 w787]
            tunnel: [w777 w784] -> w221
            tunnel: w240 -> [w775 w780]
            tunnel: w246 -> [w776 w781]
            tunnel: [w775 w779] -> w243
            frame False {
            }
            frame True {
              n177 = control-ref of="Status"() -> (w783:refnum<vi>)
              n178 = call "S2DS_READING FROM INSTRUMENTS.vi"("Status"=w783, "error in (no error)"=w786, "Data (in)"=w781, "RC info list (in)"=w780, "Instrument Info (in)"=w787) -> ("error out"=w785:errorcluster, "Data (out)"=w782:dbl[], "RC info list (out)"=w779:T8, "Instrument Info (out)"=w784:T14)
            }
          }
          n179 = case "Showing plot" shown="True" "View Plot?" {
            tunnel: w309 -> [_ w377]
            frame False {
            }
            frame True {
              n180 = property on="X axis" class="Ring (strict)"() -> ("RingText.Text"=w382:string)  [unwired: 2 in, 2 out]
              n181 = property on="Y axis" class="Ring (strict)"() -> ("RingText.Text"=w381:string)  [unwired: 2 in, 2 out]
              n182 = call "S2DS_GenerateLinePlotArray.vi"("X axis"="X axis", "Y axis"="Y axis", "Cluster in"=w377) -> ("Array"=→"XY Graph":T22)
              n183 = property on="XY Graph" class="XYGraph (strict)"("XScale.NameLbl.Text"=w382, "YScale.NameLbl.Text"=w381) -> ()  [unwired: 2 in, 2 out]
            }
          }
          n184 = Bundle By Name(cluster=w280, "Sweep ON?"=w202, "Scan type"="Scan type", "X sweep direction"="X sweep direction", "Y sweep direction"="Y sweep direction") -> (w266:T13)
          n185 = And(x=w191, y="Read array instruments") -> (x .and. y?=w294:bool)
          n186 = case "Reading and error checking of scan parameters" shown="False" "Hide control panel" {
            tunnel: [w609 w666] -> w262
            tunnel: w266 -> [w614 w666]
            tunnel: [w613 w665] -> w265
            tunnel: w267 -> [w607 w665]
            frame False {
              n187 = while {
                tunnel: w614 -> [w660]
                tunnel: [w664] -> w612
                stop <- w657 stop-if-true
                n188 = Bundle By Name(cluster=w660, "X min"="X Min", "X max"="X Max", "X bin size"="X Bin size", "X stop at"="X Stoppage", "X skip"="X Skipping", "X stopping"="X Stop at", "X data taking"="Take data") -> (w647:T13)
                n189 = call "S2DS_ErrorCheckingInX (unitless).vi"("Scan parameters in"=w647) -> ("Error string"=w663:string, "Error?"=w658:bool)
                n190 = Bundle By Name(cluster=w647, "Y min"="Y Min", "Y max"="Y Max", "Y bin size"="Y Bin size", "Y stop at"="Y Stoppage", "Y skip"="Y Skipping", "Y stopping"="Y Stop at", "Y data taking"="Take data 2") -> (w664:T13)
                n191 = call "S2DS_ErrorCheckingInY.vi"("Scan parameters in"=w664) -> ("Error string out"=w639:string, "Error? (out)"=w638:bool)
                n192 = Not Or(1:w658, 2:w638) -> (0:w657:bool)
                n193 = Concatenate Strings(w663, w639) -> (w662:string)
                n194 = Concatenate Strings("Error: " ("string"), w662) -> (w656:string)
                n195 = Select(t="", s=w657, f=w656) -> (s? t:f=→"Prameter error":string)
              }
              n196 = for {
                tunnel: w607 -> [w627] mode=indexing
                tunnel: [w623] -> w613 mode=indexing
                i -> [w631]
                n197 = case shown="0, Default" w631 {
                  tunnel: ["X Step" "Y Step"] -> w626
                  tunnel: ["X Rate up" "Y Rate up"] -> w625
                  tunnel: ["X Rate down" "Y Rate down"] -> w624
                  frame 0, Default {
                  }
                  frame 1 {
                  }
                }
                n198 = Replace Array Subset(array=w627, new element #1=w626, index #1=3 ("index"), new element #2=w625, index #2=4 ("index"), new element #3=w624, index #3=5 ("index")) -> (w623:dbl[])
              }
              n199 = case shown="True" "Reset skipped X" {
                tunnel: w612 -> [w619 w622]
                tunnel: [w619 w620] -> w610
                frame False {
                }
                frame True {
                  n200 = Bundle By Name(cluster=w622, "X reached"=0) -> (w620:T13)
                }
              }
              n201 = case shown="True" "Reset skipped Y" {
                tunnel: w610 -> [w615 w618]
                tunnel: [w615 w616] -> w609
                frame False {
                }
                frame True {
                  n202 = Bundle By Name(cluster=w618, "Y reached"=0 ("X reached")) -> (w616:T13)
                }
              }
            }
            frame True {
            }
          }
          n203 = case "Read array instruments" shown="True" w294 {
            tunnel: [w720 w726] -> w283
            tunnel: w221 -> [w720 w725]
            tunnel: [w719 w724] -> w209
            tunnel: w220 -> [w719 w723]
            tunnel: [dbl[][] [] ("Array") w722] -> w247
            tunnel: ["" ("Status") "Reading at: Array Inst" ("Status")] -> w223
            frame False {
            }
            frame True {
              n204 = call "S2DS_READ ARRAY INSTRUMENTS.vi"("error in (no error)"=w723, "Instrument Info (out) in"=w725) -> ("error out"=w724:errorcluster, "Array"=w722:dbl[][], "Instrument Info (out) out"=w726:T14)  [unwired: 1 in]
            }
          }
          n205 = case "Data analysis & sorting" shown="True" w191 {
            tunnel: w289 -> [w770 w773]
            tunnel: w235 -> [w769 w774]
            tunnel: [w770 w772] -> w245
            tunnel: [w769 w771] -> w234
            frame False {
            }
            frame True {
              n206 = call "S2DS_DataSorting.vi"("Data (in)"=w773, "DAC info list"=w774) -> ("Data (out)"=w772:dbl[], "DAC info list (out)"=w771:T10)  [unwired: 4 in]
            }
          }
          n207 = property on="Status" class="Str"("Value"=w223) -> ()  [unwired: 2 in, 2 out]
          n208 = And(x=w191, y="Export Data") -> (x .and. y?=w284:bool)
          n209 = call "S2DS_ClearBuffer.vi"("Buffer length in"=w298, "Data array in"=w215, "Clear Buffer?"="Clear Buffer?") -> ("Buffer length out"=w276:i32, "Data array out"=w278:dbl[][])  [unwired: 1 in]
          n210 = case "Data export" shown="True" w284 {
            tunnel: w245 -> [_ w762]
            tunnel: [w757 w761] -> w296
            tunnel: w295 -> [w757 w760]
            tunnel: w209 -> [w756 w759]
            tunnel: [w756 w758] -> w208
            frame False {
            }
            frame True {
              n211 = call "S2DS_Export data (SubVI).vi"("error in (no error)"=w759, "Data in"=w762, "connection id"=w760) -> ("error out"=w758:errorcluster, "connection out"=w761:refnum<k13>)  [unwired: 7 in]
            }
          }
          n212 = case "Incorporate data from array instrument" shown="True" w294 {
            tunnel: w245 -> [_ w673]
            tunnel: w247 -> [_ w672]
            tunnel: [dbl[][] [] ("2D data out") w671] -> w293
            tunnel: [w667 w670] -> w205
            tunnel: w206 -> [w667 w670]
            frame False {
            }
            frame True {
              n213 = Unbundle By Name(w670) -> ("Factors"=w669:dbl[])
              n214 = call "S2DS_Generate 2D data.vi"("2D data in"=w672, "1D data in"=w673, "Factors"=w669) -> ("2D data out"=w671:dbl[][])  [unwired: 6 in]
            }
          }
          n215 = for "Displaying data" {
            tunnel: w245 -> [w398] mode=indexing
            i -> [w399]
            n216 = case shown="14" w399 {
              tunnel: w398 -> [w400 w401 w402 w403 w404 w405 w406 w407 w408 w409 w410 w411 w412 w413 w414 w415 _]
              frame 0 {
                "X :" <- w400
              }
              frame 1 {
                "Y :" <- w401
              }
              frame 2 {
                "R0" <- w402
              }
              frame 3 {
                "R1" <- w403
              }
              frame 4 {
                "R2" <- w404
              }
              frame 5 {
                "R3" <- w405
              }
              frame 6 {
                "R4" <- w406
              }
              frame 7 {
                "R5" <- w407
              }
              frame 8 {
                "R6" <- w408
              }
              frame 9 {
                "R7" <- w409
              }
              frame 10 {
                "R8" <- w410
              }
              frame 11 {
                "R9" <- w411
              }
              frame 12 {
                "R10" <- w412
              }
              frame 13 {
                "R11" <- w413
              }
              frame 14 {
                "R12" <- w414
              }
              frame 15 {
                "R13" <- w415
              }
              frame 16, Default {
              }
            }
          }
          n217 = case "Update buffer" shown="True" w157 {
            tunnel: w278 -> [w695 w702]
            tunnel: w244 -> [_ w701]
            tunnel: [w695 w700] -> w277
            tunnel: w276 -> [w694 w699]
            tunnel: [w694 w698] -> w275
            tunnel: w214 -> [_ w697]
            tunnel: w213 -> [_ w696]
            frame False {
            }
            frame True {
              n218 = case shown="False" w696 {
                tunnel: w702 -> [w703 _]
                tunnel: w701 -> [w705 _]
                tunnel: [w704 w706] -> w700
                tunnel: w697 -> [_ w706]
                frame False {
                  n219 = Build Array (concatenate)(w703, w705) -> (w704:dbl[][])
                }
                frame True {
                }
              }
              n220 = Increment(x=w699) -> (x+1=w698:i32)
            }
          }
          n221 = Unbundle By Name(w196) -> ("Buffer size"=w203:i32)
          n222 = Select(t=1, s=w213, f=w203) -> (s? t:f=w270:i32)
          n223 = Greater Or Equal?(x=w275, y=w270) -> (x >= y?=w272:bool)
          n224 = Compound Arithmetic op=OR(w169, "Save now to file?", w272, w281) -> (w273:bool)
          n225 = case "Save to file" shown="True" w273 {
            tunnel: [w708 w716] -> w242
            tunnel: [w709 w713] -> w307
            tunnel: w277 -> [w709 w714]
            tunnel: w197 -> [w708 w715]
            tunnel: w275 -> [w707 w711]
            tunnel: [w707 w712] -> w299
            frame False {
            }
            frame True {
              n226 = call "S2DS_Writing buffer to file.vi"("Data save info (in)"=w715, "Data array in"=w714, "Buffer length"=w711) -> ("Data save info (out)"=w716:T3, "Data array out"=w713:dbl[][], "Buffer length out"=w712:i32)  [unwired: 4 in]
              n227 = property on="Save now to file?" class="Bool (strict)"("Value"=FALSE ("Save now to file?")) -> ()  [unwired: 2 in, 2 out]
            }
          }
          "Buffer length:" <- w299
          n228 = And(x=w158, y="External control") -> (x .and. y?=w286:bool)
          n229 = case shown="True" "Pause" {
            frame False {
            }
            frame True {
              n230 = flat-sequence {
                frame #0 {
                  n231 = while {
                    stop <- w729 continue-if-true
                    n232 = Wait (ms)(milliseconds to wait=u32 100) -> ()  [unwired: 1 out]
                    n233 = property on="Status" class="Str"("Value"="Paused by User" ("Status"), "Text.TextColor"=u32 16711680) -> ()  [unwired: 2 in, 2 out]
                    n234 = property on="Pause" class="Bool (strict)"() -> ("Value"=w729:bool)  [unwired: 2 in, 2 out]
                  }
                }
                frame #1 {
                  n235 = property on="Status" class="Str"("Value"="" ("Status"), "Text.TextColor"=u32 32639) -> ()  [unwired: 2 in, 2 out]
                }
              }
            }
          }
          n236 = case "External control" shown="True" w286 {
            tunnel: w208 -> [w764 w768]
            tunnel: [w764 w767] -> w288
            tunnel: w211 -> [w763 w766]
            tunnel: [w763 w766] -> w297
            frame False {
            }
            frame True {
              n237 = call "S2DS_External Control (SubVI).vi"("error in (no error)"=w768, "Timeout (ms), Check interval (ms)"=w766) -> ("error out"=w767:errorcluster)  [unwired: 9 in]
              n238 = property on="Status" class="Str"("Value"="Waiting for external response" ("Status")) -> ()  [unwired: 2 in, 2 out]
            }
          }
          n239 = case "Decision maker: Decide next scan parameters (e.g. X-Y target)" shown="False" "Ramping" {
            tunnel: w280 -> [w540 _]
            tunnel: [w551 w602] -> w162
            tunnel: w262 -> [w548 w603]
            tunnel: [w550 FALSE ("Change  x direction")] -> w264
            tunnel: [w549 FALSE ("Change y direction")] -> w263
            tunnel: w190 -> [w544 _]
            tunnel: [w543 FALSE ("WC from file?")] -> w167
            frame False {
              n240 = Unbundle By Name(w548) -> ("X reached"=→"X reached":i32, "Y reached"=→"Y reached":i32)
              n241 = Unbundle By Name(w548) -> ("Sweep ON?"=w539:bool, "Scan type"=w542:i32)
              n242 = case shown="True" w539 {
                tunnel: w540 -> [_ w561]
                tunnel: [w556 w565] -> w551
                tunnel: w548 -> [w556 w564]
                tunnel: [FALSE ("Change  x direction") w563] -> w550
                tunnel: [FALSE ("Change y direction") w562] -> w549
                tunnel: [w553 w559] -> w545
                tunnel: w544 -> [_ w560]
                tunnel: [w553 w559] -> w541
                tunnel: [FALSE ("WC from file?") w557] -> w543
                tunnel: w542 -> [_ w558]
                frame False {
                  w553 = T2."Enabled" ("Disabled")
                }
                frame True {
                  w559 = T2."Disabled and Grayed Out" ("Disabled")
                  n243 = case shown="1, Default" w558 {
                    tunnel: [w585 w600] -> w565
                    tunnel: w564 -> [w581 w600]
                    tunnel: [w577 FALSE ("Change  x direction")] -> w563
                    tunnel: [w576 FALSE ("Change y direction")] -> w562
                    tunnel: w561 -> [w567 _]
                    tunnel: w560 -> [w573 _]
                    tunnel: [FALSE TRUE] -> w557
                    frame 1, Default {
                      n244 = call "S2DS_CheckingScanOverInX.vi"("Scan parameters in (old)"=w567, "Scan parameters in (new)"=w581) -> ("Scan parameters out"=w580:T13)
                      n245 = Unbundle By Name(w567) -> ("Sweep ON?"=w566:bool)
                      n246 = call "S2DS_CheckingScanOverInY.vi"("Scan parameters in (old)"=w567, "Scan parameters in (new)"=w580) -> ("Scan parameters out"=w582:T13)
                      n247 = property on="Script On?" class="Bool (strict)"("DisabledEnum"=T2."Enabled" ("Disabled")) -> ()  [unwired: 2 in, 2 out]
                      n248 = Unbundle By Name(w582) -> ("Sweep ON?"=w583:bool)
                      n249 = property on="Script On?" class="Bool (strict)"() -> ("Value"=w571:bool)  [unwired: 2 in, 2 out]
                      n250 = Not(x=w571) -> (.not. x?=w570:bool)
                      n251 = call "S2DS_Core decision-New.vi"("Ramp X"="Ramp X", "Ramp Y"="Ramp Y", "Scan parameters out  in"=w582, "Sweep ON?"=w583) -> ("Turn off Sweep?"=w574:bool, "Sweep Over?"=w569:bool, "Scan parameters out"=w584:T13)  [unwired: 5 in]
                      n252 = And(x=w570, y=w569) -> (x .and. y?=w572:bool)
                      n253 = case shown="True" w574 {
                        selector: w574 -> [w596 _]
                        frame False {
                          n254 = property on="Sweep" class="Bool (strict)"("Value"=w596) -> ()  [unwired: 2 in, 2 out]
                        }
                        frame True {
                        }
                      }
                      n255 = case shown="True" w566 {
                        tunnel: [w588 w594] -> w585
                        tunnel: w584 -> [w588 w593]
                        tunnel: [FALSE ("Change  x direction") w592] -> w577
                        tunnel: [FALSE ("Change y direction") w591] -> w576
                        tunnel: w573 -> [_ w589]
                        frame False {
                        }
                        frame True {
                          n256 = call "S2DS_DetermineTargetInX.vi"("Measurement ON?"=w589, "Scan parameters  in"=w593) -> ("Change  x direction"=w592:bool, "Scan parameters  out"=w590:T13)
                          n257 = call "S2DS_DetermineTargetInY.vi"("Measurement ON?"=w589, "Scan parameters  in"=w590) -> ("Change y direction"=w591:bool, "Scan parameters  out"=w594:T13)
                        }
                      }
                      n258 = case shown="True" w572 {
                        frame False {
                        }
                        frame True {
                          n259 = property on="Send email" class="Bool (strict)"() -> ("Value"=w595:bool)  [unwired: 2 in, 2 out]
                          n260 = call "S2DS_Pop-Up Message.vi"("Send mail?"=w595) -> ()  [unwired: 11 in]
                        }
                      }
                    }
                    frame 0 {
                    }
                  }
                }
              }
              n261 = property on="Edit Instrument?" class="Bool"("DisabledEnum"=w545) -> ()  [unwired: 2 in, 2 out]
              n262 = property on="Scan type" class="Ring (strict)"("DisabledEnum"=w541) -> ()  [unwired: 2 in, 2 out]
            }
            frame True {
              n263 = call "S2DS_Ramp or Go to (SubVI).vi"("Scan parameters in"=w603) -> ("Scan parameters out"=w602:T13)  [unwired: 10 in]
              n264 = property on="Sweep" class="Bool (strict)"("Value"=FALSE) -> ()  [unwired: 2 in, 2 out]
            }
          }
          n265 = Unbundle By Name(w280) -> ("Scan type"=w256:i32, "Sweep ON?"=w260:bool)
          n266 = Unbundle By Name(w262) -> ("Scan type"=w255:i32, "Sweep ON?"=w248:bool)
          n267 = Not Equal?(x=w260, y=w248) -> (x != y?=w258:bool)
          n268 = Not Equal?(x=w256, y=w255) -> (x != y?=w254:bool)
          n269 = Compound Arithmetic op=OR("Timer reset?", w258, w254) -> (w257:bool)
          n270 = case shown="True" w248 {
            tunnel: [w522 w533] -> w312
            tunnel: w310 -> [w522 w532]
            tunnel: w262 -> [_ w531]
            tunnel: w257 -> [_ w530]
            tunnel: w226 -> [_ w526]
            tunnel: w168 -> [_ w523]
            frame False {
            }
            frame True {
              n271 = call "S2DS_Timer.vi"("Timer reset?"=w530, "WC read from file info (out)"=w523, "Scan parameters"=w531, "Timer Cluster in"=w532) -> ("Progress"=→"Progress":i32, "Remaining time"=w527:dbl, "Elapsed time"=w528:dbl, "Timer Cluster out"=w533:T20)  [unwired: 1 in]
              n272 = Quotient & Remainder(x=w526, y=10) -> (x-y*floor(x/y)=w524:i32)  [unwired: 1 out]
              n273 = case shown="0" w524 {
                tunnel: w528 -> [_ w537]
                tunnel: w527 -> [_ w536]
                frame 1, Default {
                }
                frame 0 {
                  w538 = "%t"
                  n274 = Format Into String(format string=w538, w537) -> (resulting string=→"Elapsed time:":string)  [unwired: 2 in, 1 out]
                  n275 = Format Into String(format string=w538, w536) -> (resulting string=→"Remaining time: :":string)  [unwired: 2 in, 1 out]
                }
              }
            }
          }
          n276 = call "S2DS_Update X Y Channel from scan parameters.vi"("Scan parameters in"=w162, "WC info in"=w230, "Write channel parameters (in)"=w265) -> ("WC info out"=w178:T6)  [unwired: 8 in]
          n277 = case shown="True" w167 {
            tunnel: w178 -> [w337 w346]
            tunnel: [w337 w347] -> w172
            tunnel: [w338 w345] -> w177
            tunnel: w161 -> [w338 _]
            tunnel: [w336 w344] -> w176
            tunnel: w168 -> [w336 w343]
            tunnel: [FALSE ("File over?") w342] -> w174
            tunnel: w162 -> [_ w341]
            frame False {
            }
            frame True {
              n278 = property on="Ramp X" class="Bool (strict)"() -> ("Value"=w340:bool)  [unwired: 2 in, 2 out]
              n279 = property on="Ramp Y" class="Bool (strict)"() -> ("Value"=w339:bool)  [unwired: 2 in, 2 out]
              n280 = call "S2DS_WCFromFile.vi"("Ramp Y to zero?"=w339, "Ramp X to zero?"=w340, "Scan parameters in"=w341, "WC read from file info (in)"=w343, "WC info list in"=w346) -> ("Index"=w345:i32, "WC read from file info (out)"=w344:T19, "WC info list out"=w347:T6, "File over?"=w342:bool)  [unwired: 2 in, 1 out]
            }
          }
          n281 = control-ref of="Status"() -> (w290:refnum<vi>)
          n282 = control-ref of="Y sweep direction"() -> (w170:refnum<vi>)
          n283 = case shown="True" "WC calculation" {
            tunnel: w172 -> [w348 w351]
            tunnel: [w348 w350] -> w184
            tunnel: w181 -> [_ w349]
            frame False {
            }
            frame True {
              n284 = call "S2DS_ComputeWC.vi"("Parsed Formula Node"=w349, "WC info in"=w351) -> ("WC info out"=w350:T6)  [unwired: 8 in, 1 out]
            }
          }
          n285 = call "S2DS_WRITING TO INSTRUMENTS.vi"("Index"=w177, "Timeout (s)"="Timeout", "error in"=w288, "Status refnum"=w290, "WC info in"=w184, "Instrument Info (in)"=w283) -> ("error out"=w292:errorcluster, "Data out"=w308:dbl[], "WC info out"=w204:T6, "Instrument Info (out)"=w311:T14)
          n286 = control-ref of="X sweep direction"() -> (w171:refnum<vi>)
          n287 = case shown="False" w167 {
            tunnel: [w323 w326] -> w306
            tunnel: [w322 w331] -> w304
            tunnel: [w321 w331] -> w303
            tunnel: [w320 w324] -> w302
            tunnel: w264 -> [w319 _]
            tunnel: w263 -> [w318 _]
            tunnel: w162 -> [w317 w328]
            tunnel: [w316 w327] -> w193
            tunnel: w174 -> [_ w324]
            tunnel: TRUE ("Measurement") -> [w315 w331]
            tunnel: w172 -> [_ w325]
            tunnel: w171 -> [w314 w330]
            tunnel: w170 -> [w313 w329]
            frame False {
              n288 = call "S2DS_Change direction.vi"("X sweep direction"=w314, "Y sweep direction"=w313, "Change y direction?"=w318, "Change x direction?"=w319, "Scan parameters  in"=w317) -> ("Scan over?"=w320:bool, "Scan parameters out"=w316:T13, "Change color"=w323:bool)  [unwired: 3 in]
              n289 = call "S2DS_ConditionForWriteToBufferNew.vi"("Measurement"=w315, "Scan parameters in"=w316) -> ("Update on?"=w321:bool, "Measurement on?"=w322:bool)  [unwired: 3 in]
            }
            frame True {
              n290 = case shown="False" w324 {
                frame False {
                }
                frame True {
                  n291 = property on="Script On?" class="Bool (strict)"() -> ("Value"=w332:bool)  [unwired: 2 in, 2 out]
                  n292 = property on="Sweep" class="Bool (strict)"("Value"=FALSE ("Sweep")) -> ()  [unwired: 2 in, 2 out]
                  n293 = case shown="False" w332 {
                    frame False {
                      n294 = property on="Send email" class="Bool (strict)"() -> ("Value"=w334:bool)  [unwired: 2 in, 2 out]
                      n295 = call "S2DS_Pop-Up Message.vi"("Send mail?"=w334) -> ()  [unwired: 11 in]
                    }
                    frame True {
                    }
                  }
                }
              }
              n296 = call "S2DS_Change directionWCFromFile.vi"("WC info list in"=w325, "Scan parameters  in"=w328, "Y sweep direction"=w329, "X sweep direction"=w330) -> ("Scan parameters out"=w327:T13, "Change color"=w326:bool)  [unwired: 5 in]
            }
          }
          n297 = case shown="False" "Quit sweep" {
            selector: "Quit sweep" -> [w394 _]
            tunnel: [w394 w395] -> w301
            tunnel: w193 -> [_ w396]
            frame False {
            }
            frame True {
              n298 = property on="Buffer length:" class="DigNum (strict)"() -> ("Value"=w397:i32)  [unwired: 2 in, 2 out]
              n299 = call "S2DS_ExitCondition.vi"("Scan parameters in"=w396, "Buffer length"=w397) -> ("Yes, exit."=w395:bool)  [unwired: 7 in]
            }
          }
        }
      }
    }
    "Status" <- "Back panel not set" ("Status")
  }
